vi "Open Project Ref.vi"(8 "error in (no error)":errorcluster, 10 "Project Path":path) -> (0 "error out":errorcluster, 2 "Project Ref out":refnum<vi>)   [LabVIEW 2019, in "Project Sync Tools.lvclass"]
uses:
  Project Sync Tools.lvclass
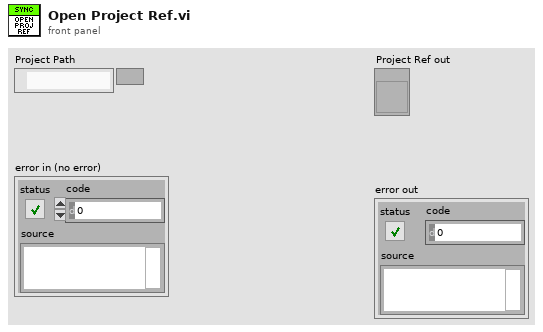
[diagram p1: front panel]
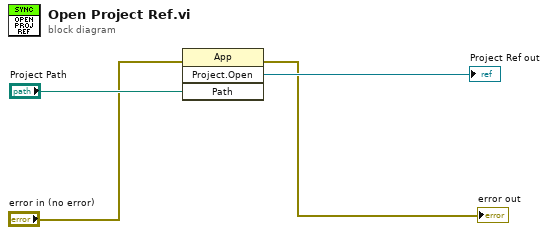
[diagram p0: block diagram]
diagram:
  n1 = invoke class="App" method="Project.Open"(error in="error in (no error)", "Path"="Project Path") -> (error out=→"error out":errorcluster, "Project:Open"=→"Project Ref out":refnum<vi>)  [unwired: 2 in, 2 out]
